vi "Step Check.vi"(1 "Step":dbl, 2 "New Value":dbl, 3 "Old Value":dbl) -> (0 "Instant output":bool)   [LabVIEW 2013]
doc: "Если изменение меньше 5 шагов, выводим новое значение сразу, если больше, то плавно"
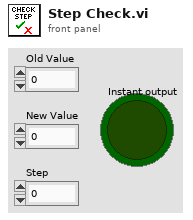
[diagram p1: front panel]
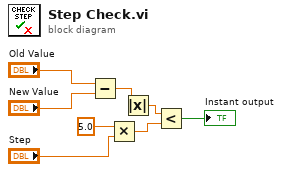
[diagram p0: block diagram]
diagram:
  n1 = Subtract(x="Old Value", y="New Value") -> (x-y=w2:dbl)
  n2 = Multiply(x=5.0, y="Step") -> (x*y=w6:dbl)
  n3 = Absolute Value(x=w2) -> (abs(x)=w3:dbl)
  n4 = Less?(x=w3, y=w6) -> (x < y?=→"Instant output":bool)
